vi "ServoHostArm.vi"(8 "error in":errorcluster, 9 "Angle (deg) Arm":dbl(slide) scale=-90.0..90.0, 11 "FPGA VI Reference In":T1) -> (0 "error out":errorcluster, 3 "FPGA VI Reference Out 2":T1)   [LabVIEW 2012]
uses:
  FPGA_ref.ctl
  <vilib>/Utility/error.llb/Error Cluster From Error Code.vi
  <vilib>/rvi/errors/niLvFpgaAdjustHostInterfaceError.vi
  <vilib>/rvi/interface/nirviReadWriteControl/nirviReadWriteControl.xnode
  NiFpgaLv.dll
  <vilib>/rvi/interface/Simulation/niFpgaSimulationCallBeginRW.vi
panel:
  in  "lower limit (arm)":dbl=-89.0
  in  "upper limit (Arm)":dbl=51.0
  out "pulse width (us)":i32
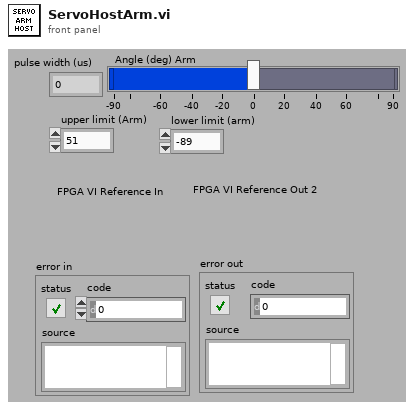
[diagram p1: front panel]
types:
  T1 = typedef "FPGA_ref.ctl" = refnum<k20>
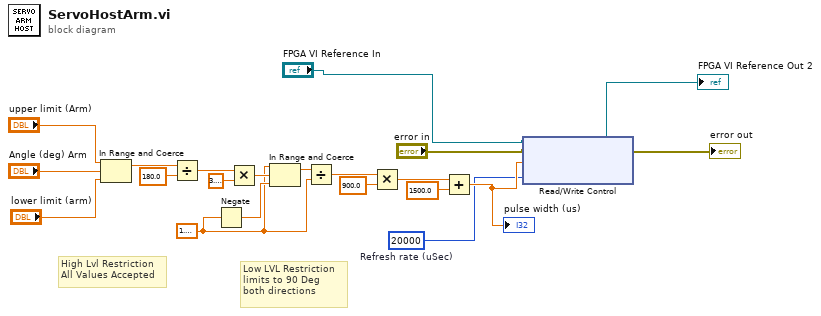
[diagram p0: block diagram]
diagram:
  w10 = 1.5707963267948966
  w1 = u32 20000  # Refresh rate (uSec)
  # "Low LVL Restriction\nlimits to 90 Deg \nboth directions"
  # "High Lvl Restriction\nAll Values Accepted"
  n1 = In Range and Coerce(upper limit="upper limit (Arm)", x="Angle (deg) Arm", lower limit="lower limit (arm)") -> (coerced(x)=w11:dbl)  [unwired: 1 out]
  n2 = Divide(x=w11, y=180.0) -> (x/y=w15:dbl)
  n3 = Negate(x=w10) -> (-x=w16:dbl)
  n4 = Multiply(x=w15, y=3.141592653589793) -> (x*y=w14:dbl)
  n5 = In Range and Coerce(upper limit=w10, x=w14, lower limit=w16) -> (coerced(x)=w17:dbl)  [unwired: 1 out]
  n6 = Divide(x=w17, y=w10) -> (x/y=w18:dbl)
  n7 = Multiply(x=w18, y=900.0) -> (x*y=w20:dbl)
  n8 = Add(x=w20, y=1500.0) -> (x+y=w2:dbl)
  "pulse width (us)" <- w2
  n9 = xnode "Read/Write Control"("FPGA VI Reference In"="FPGA VI Reference In", "error in"="error in", "servo Arm"=w2, "Count(uSec) Arm"=w1) -> ("FPGA VI Reference Out"=→"FPGA VI Reference Out 2":T1, "error out"=→"error out":errorcluster)
